vi "ELVIS III v1.0 Build Mutex Name.vi"(10 "Mutex ID":i32, 11 "Connector":T1=enum."ConnectorB") -> (3 "Mutex Name":string)   [LabVIEW 2021]
uses:
  <vilib>/myRIO/Common/Instrument Driver Framework/ELVIS III v1.0/Resource Manager/typedefs/ELVIS III v1.0 Connector List.ctl
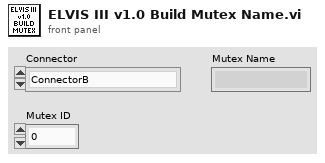
[diagram p1: front panel]
types:
  T1 = typedef "ELVIS III v1.0 Connector List.ctl" = enum32{"None", "ConnectorA", "ConnectorB"}
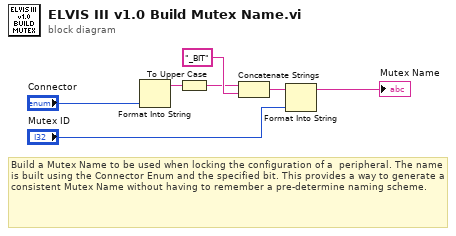
[diagram p0: block diagram]
diagram:
  # "Build a Mutex Name to be used when locking the configuration of a  peripheral. The name is built using the Connector Enum and the specified bit. This provides a way to generate a consistent Mutex Name without having to remember a pre-determine naming scheme."
  n1 = Format Into String("Connector") -> (resulting string=w3:string)  [unwired: 3 in, 1 out]
  n2 = To Upper Case(1:w3) -> (0:w2:string)
  n3 = Concatenate Strings(w2, "_BIT" ("string")) -> (w1:string)
  n4 = Format Into String(initial string=w1, "Mutex ID") -> (resulting string=→"Mutex Name":string)  [unwired: 2 in, 1 out]
